vi "Pixel to Vertical Angle Offset.vi"(11 "Pixel on level with camera":dbl=200.0) -> (3 "Vertical Angle Offset":dbl=6.75)   [LabVIEW 2012]
panel:
  in  "Vertical Field of View":dbl=54.0
  in  "Vertical Resolution":dbl=320.0
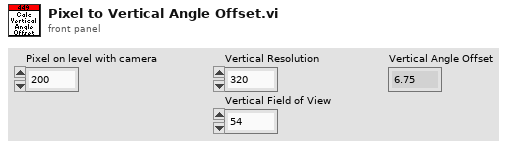
[diagram p1: front panel]
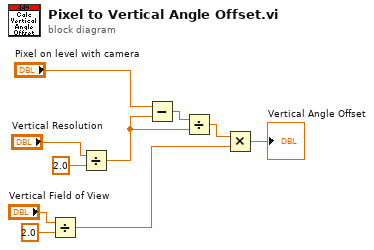
[diagram p0: block diagram]
diagram:
  n1 = Divide(x="Vertical Field of View", y=2.0) -> (x/y=w2:dbl)
  n2 = Divide(x="Vertical Resolution", y=2.0) -> (x/y=w6:dbl)
  n3 = Subtract(x="Pixel on level with camera", y=w6) -> (x-y=w7:dbl)
  n4 = Divide(x=w7, y=w6) -> (x/y=w5:dbl)
  n5 = Multiply(x=w5, y=w2) -> (x*y=→"Vertical Angle Offset":dbl)
